vi "ATA10003-ONOFF.vi"(7 "Delay Time (s)":dbl=0.5, 8 "error in":errorcluster caption="错误输入（无错误）", 9 "OutputCtrl":bool, 10 "Address(0x01)":u8=1 format="%.0x", 11 "MyIndex":u8) -> (0 "error out":errorcluster, 3 "Result":bool)   [LabVIEW 2015]
uses:
  <vilib>/Instr/_visa.llb/VISA Configure Serial Port (Instr).vi
panel:
  out "VISA":refnum<visa-resource-name>
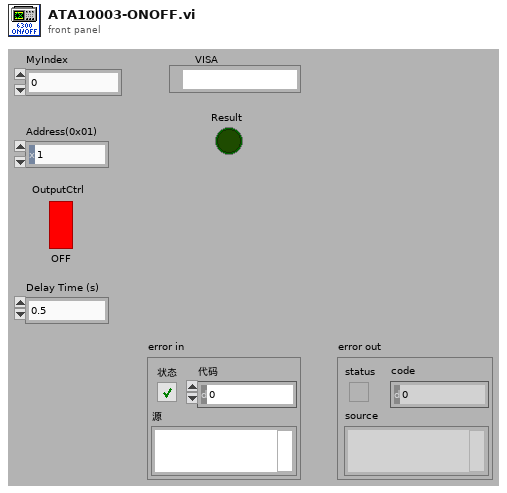
[diagram p1: front panel]
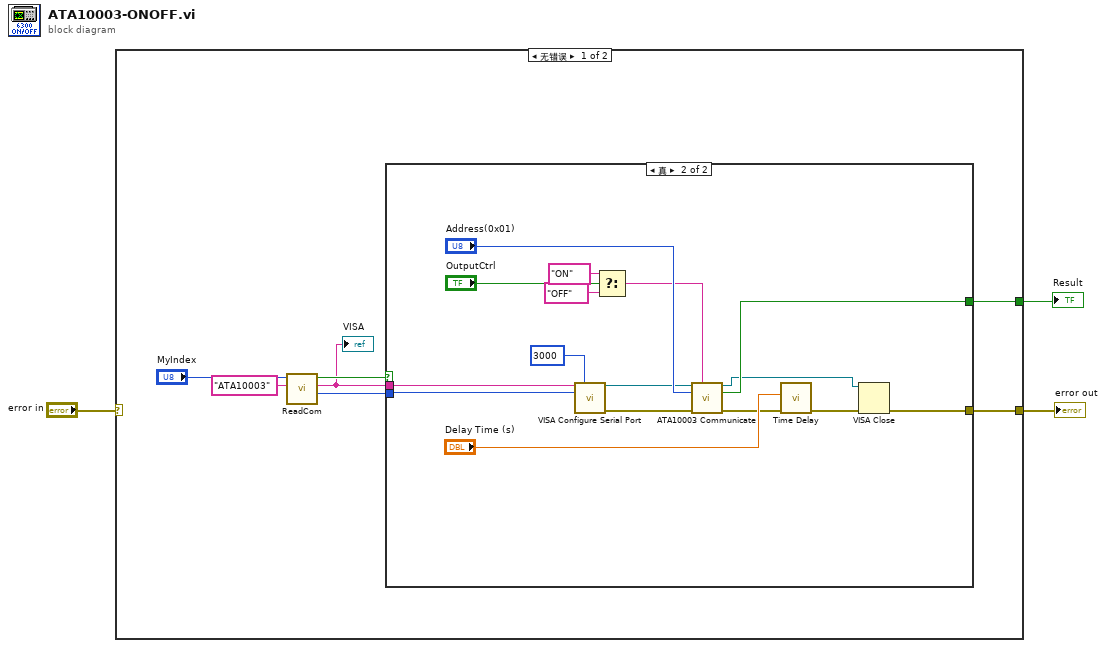
[diagram p0: block diagram]
diagram:
  n1 = case shown="无错误" "error in" {
    selector: "error in" -> [_ w27]
    tunnel: [w10 _] -> w3
    tunnel: [w4 w27] -> w2
    frame No Error {
      n2 = call "ReadCom.vi"("仪器名称"="ATA10003", "MyIndex"="MyIndex") -> ("Baudrate"=w6:i32, "COM"=w5:string, "OK?"=w7:bool)  [unwired: 7 in]
      "VISA" <- w5
      n3 = case shown="真" w7 {
        tunnel: [_ w26] -> w10
        tunnel: w5 -> [_ w15]
        tunnel: w6 -> [_ w14]
        tunnel: [_ w12] -> w4
        frame False {
        }
        frame True {
          n4 = call-poly "VISA Configure Serial Port"("VISA resource name"=w15, "timeout (10sec)"=u32 3000, "baud rate (9600)"=w14) -> ("VISA resource name out"=w17:refnum<visa-resource-name>, "error out"=w16:errorcluster)  [unwired: 11 in]
          n5 = Select(t="ON" ("Function_In"), s="OutputCtrl", f="OFF" ("Function_In")) -> (s? t:f=w18:string)
          n6 = call "ATA10003 Communicate.vi"("VISA Resource In"=w17, "Function_In"=w18, "Address(0x01)"="Address(0x01)", "error in (no error)"=w16) -> ("VISA Resource Out"=w13:refnum<visa-resource-name>, "OK ?"=w26:bool, "error out"=w21:errorcluster)  [unwired: 7 in, 2 out]
          n7 = call "Time Delay"("error in (no error)"=w21, "Delay Time (s)"="Delay Time (s)") -> ("error out"=w24:errorcluster)  [unwired: 9 in]
          n8 = VISA Close(VISA resource name=w13, error in (no error)=w24) -> (error out=w12:errorcluster)
        }
      }
    }
    frame Error {
    }
  }
  "Result" <- w3
  "error out" <- w2
